vi "Route_Switch.vi"(8 "error in (no error)":errorcluster, 10 "Parameters":string, 11 "reference in":refnum<class "Test_Flux_Capacitor.lvclass">) -> (0 "error out":errorcluster, 2 "Result":bool, 3 "reference out":refnum<class "Test_Flux_Capacitor.lvclass">)   [LabVIEW 2022 SP3, in "Test_Flux_Capacitor.lvlib" / "Test_Flux_Capacitor.lvclass"]
uses:
  Test_Flux_Capacitor.lvclass
  ParameterTypes/Connect_LCR.ctl
  <vilib>/Utility/error.llb/Trim Whitespace One-Sided.vi
  Components/SwitchBase.lvlibp/SwitchBase.lvclass
  <vilib>/JDP Science/JSONtext/JSONtext.lvlib
panel:
  in  "State":bool
  in  "Parameter_Type":T1
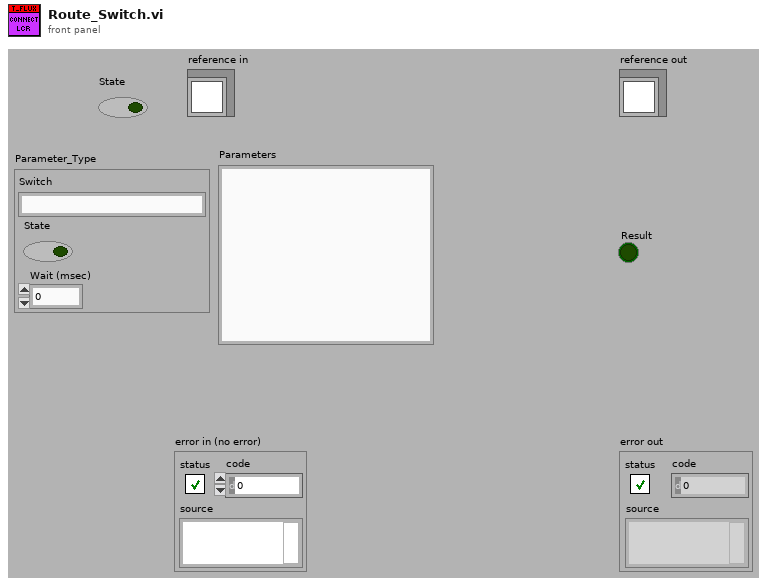
[diagram p1: front panel]
types:
  T1 = typedef "Test_Flux_Capacitor.lvlib/Test_Flux_Capacitor.lvclass/Connect_LCR.ctl" = cluster{"Switch":string, "State":bool, "Wait (msec)":u32}
  T2 = typedef "Test_Flux_Capacitor.lvlib/Test_Flux_Capacitor.lvclass/ObjectAttributes.ctl" = cluster{"Config":T3, "DMM":refnum<class "DMM_Keysight_34980A.lvclass">, "LCR":refnum<class "LCR_BK891.lvclass">, "PSU":refnum<class "PSU_Base.lvclass">, "Switch_Manager":refnum<class "SwitchBase.lvclass">, "FRAM":string, "Flux_Capacitor":refnum<class "Flux_Capacitor.lvclass">, "Frequency_Counter":refnum<class "Frequency_Counter_Base.lvclass">, "JTAG":refnum<class "JTAG_Base.lvclass">}
  T3 = typedef "Test_Flux_Capacitor.lvlib/Test_Flux_Capacitor.lvclass/Config.ctl" = cluster{"default":string}
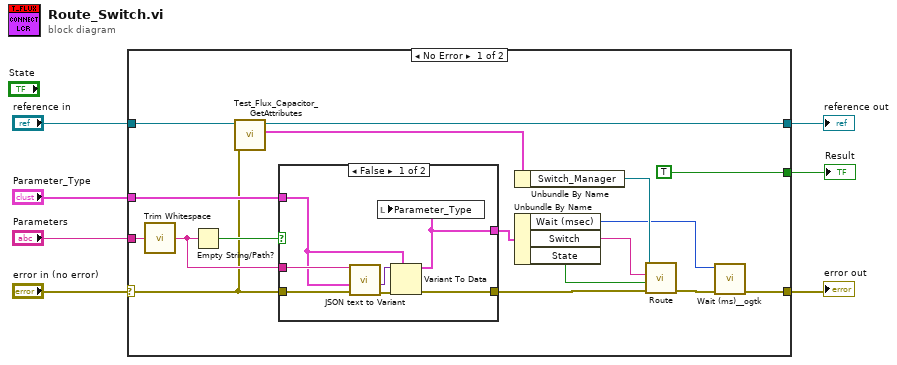
[diagram p0: block diagram]
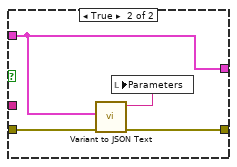
[diagram p2: hidden frame]
diagram:
  n1 = case shown="No Error" "error in (no error)" {
    selector: "error in (no error)" -> [w8 w37]
    tunnel: [w16 w37] -> w6
    tunnel: [w23 w36] -> w4
    tunnel: "reference in" -> [w24 w36]
    tunnel: "Parameters" -> [w12 _]
    tunnel: "Parameter_Type" -> [w13 _]
    tunnel: [TRUE _] -> w1
    frame No Error {
      n2 = call <vilib>:"Trim Whitespace.vi"("string"=w12) -> ("trimmed string"=w15:string)  [unwired: 1 in]
      n3 = Empty String/Path?(string/path=w15) -> (empty?=w14:bool)
      n4 = call "Test_Flux_Capacitor_GetAttributes.vi"("error in (no error)"=w8, "reference in"=w24) -> ("Data"=w22:T2, "reference out"=w23:refnum<class "Test_Flux_Capacitor.lvclass">)  [unwired: 6 in, 2 out]
      n5 = case shown="False" w14 {
        tunnel: w8 -> [w29 w34]
        tunnel: w13 -> [w25 w35]
        tunnel: [w31 w32] -> w11
        tunnel: [w30 w35] -> w10
        tunnel: w15 -> [w28 _]
        frame False {
          n6 = call <vilib>:"JSON text to Variant.vi"("error in (no error)"=w29, "Data Type"=w25, "JSON"=w28) -> ("error out"=w26:errorcluster, "Variant out"=w27:variant)  [unwired: 7 in]
          n7 = Variant To Data(error in=w26, type=w25, Variant=w27) -> (data=w30:T1, error out=w31:errorcluster)
          n8 = local write "Parameter_Type"(w30) -> ()
        }
        frame True {
          n9 = call <vilib>:"Variant to JSON Text.vi"("error in (no error)"=w34, "Variant"=w35) -> ("error out"=w32:errorcluster, "<JSON>"=w33:string)  [unwired: 7 in, 1 out]
          n10 = local write "Parameters"(w33) -> ()
        }
      }
      n11 = Unbundle By Name(w22) -> ("Switch_Manager"=w21:refnum<class "SwitchBase.lvclass">)
      n12 = Unbundle By Name(w10) -> ("Wait (msec)"=w18:u32, "Switch"=w20:string, "State"=w9:bool)
      n13 = call-dynamic "Route.vi"("error in (no error)"=w11, "Connect"=w9, "channel 1"=w20, "reference in"=w21) -> ("error out"=w19:errorcluster)  [unwired: 6 in, 1 out]
      n14 = call <userlib>:"Wait (ms)__ogtk.vi"("error in (no error)"=w19, "milliseconds to wait"=w18) -> ("error out"=w16:errorcluster)  [unwired: 8 in, 1 out]
    }
    frame Error {
    }
  }
  "Result" <- w1
  "error out" <- w6
  "reference out" <- w4
